vi "Feeder_Globals.vi"() -> ()   [LabVIEW 2020]
uses:
  Systems/Feeder/Feeder_Cluster.ctl
  Systems/Feeder/Feeder_Control_States.ctl
panel:
  in  "Funnel_Load_%Vbus":dbl=0.7
  in  "Intake_Load_%Vbus":dbl=0.5
  in  "Magazine_Load_%Vbus":dbl=0.3
  in  "Feeder_Determiner_Notifier":refnum<notifier>
  in  "Feeder_Determiner_Ref":string="Feeder_Determiner_Ref"
  # "AUTO:"
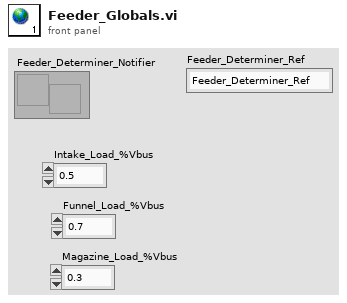
[diagram p1: front panel]
diagram:
